vi "Initialize.vi"(8 "error in (no error)":errorcluster, 10 "DM-SetPower-Command-Initialize":T1 {"Power" scale=-1.0..1.0}, 11 "DM-SetPower-Command in":refnum<class "DM-SetPower-Command.lvclass">) -> (0 "error out":errorcluster, 3 "DM-SetPower-Command out":refnum<class "DM-SetPower-Command.lvclass">)   [LabVIEW 2013, in "DM-SetPower-Command.lvclass"]
uses:
  DM-SetPower-Command.lvclass
  DM-SetPower-Command-Arguments.ctl
  States/DM-MaintainPower-State/DM-MaintainPower-State.lvclass
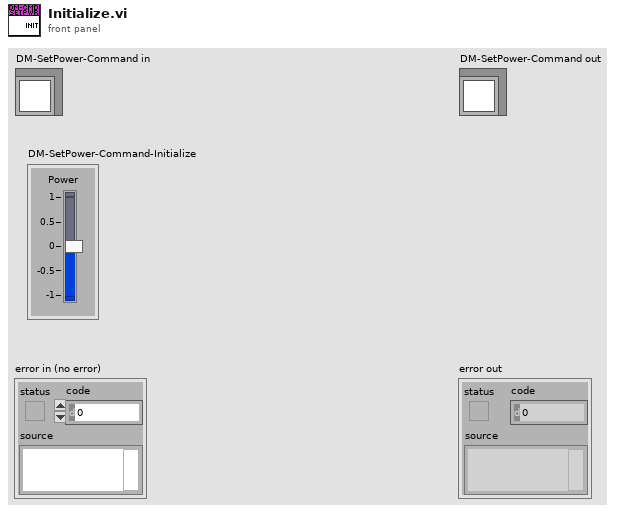
[diagram p1: front panel]
types:
  T1 = typedef "DM-SetPower-Command.lvclass/DM-SetPower-Command-Arguments.ctl" = cluster{"Power":dbl}
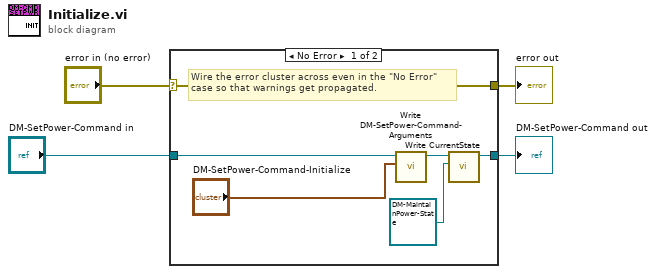
[diagram p0: block diagram]
diagram:
  n1 = case shown="No Error" "error in (no error)" {
    selector: "error in (no error)" -> [w10 w12]
    tunnel: [w10 w12] -> w3
    tunnel: [w6 w11] -> w1
    tunnel: "DM-SetPower-Command in" -> [w9 w11]
    frame No Error {
      # "Wire the error cluster across even in the \"No Error\"\ncase so that warnings get propagated."
      n2 = call-dynamic "Write DM-SetPower-Command-Arguments.vi"("DM-SetPower-Command-Initial"="DM-SetPower-Command-Initialize", "DM-SetPower-Command in"=w9) -> ("DM-SetPower-Command out"=w7:refnum<class "DM-SetPower-Command.lvclass">)  [unwired: 8 in, 1 out]
      n3 = call-dynamic "Write CurrentState.vi"("State.lvclass"=refnum<class "DM-MaintainPower-State.lvclass"> refnum ("DM-MaintainPower-State.lvclass"), "Command in"=w7) -> ("Command out"=w6:refnum<class "DM-SetPower-Command.lvclass">)  [unwired: 8 in, 1 out]
    }
    frame Error {
    }
  }
  "error out" <- w3
  "DM-SetPower-Command out" <- w1
